vi "Filter VIs to Measure.vi"(8 "error in (no error)":errorcluster, 10 "VI Paths":path[](array[path]), 11 "Coverage Analyzer in":refnum<class "Coverage Analyzer.lvclass">) -> (0 "error out":errorcluster, 2 "Filtered VI Paths":path[](array[path]), 3 "Coverage Analyzer out":refnum<class "Coverage Analyzer.lvclass">)   [LabVIEW 2020, in "Coverage Analyzer.lvlib" / "Coverage Analyzer.lvclass"]
uses:
  Coverage Analyzer.lvclass
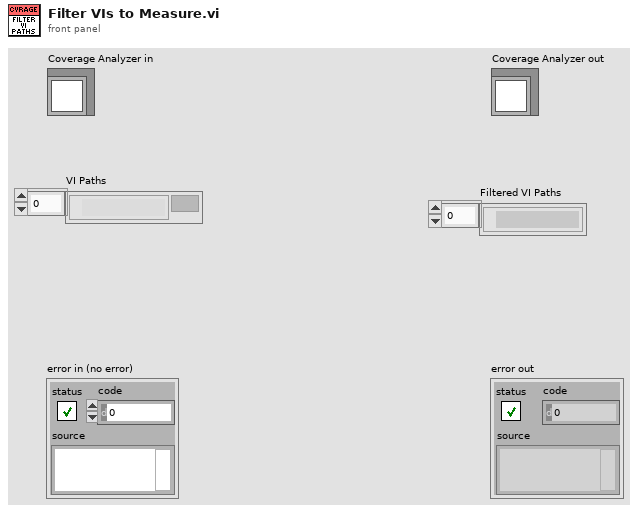
[diagram p1: front panel]
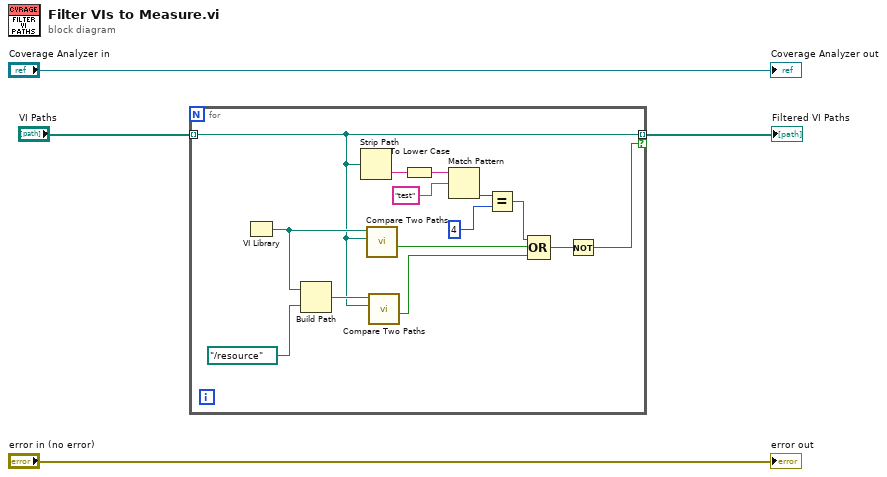
[diagram p0: block diagram]
diagram:
  n1 = for {
    tunnel: "VI Paths" -> [w11] mode=indexing
    tunnel: [w11] -> w2 mode=indexing if=w15
    n2 = VI Library() -> (path=w14:path)
    n3 = Build Path(base path=w14, name or relative path=path "../resource" ("search string")) -> (appended path=w17:path)
    n4 = Strip Path(path=w11) -> (name=w10:string)  [unwired: 1 out]
    n5 = call <vilib>:"Compare Two Paths.vi"("Path 2"=w11, "Path 1"=w14) -> ("Path 2 Relative to Path 1?"=w16:bool)  [unwired: 6 in, 3 out]
    n6 = call <vilib>:"Compare Two Paths.vi"("Path 2"=w11, "Path 1"=w17) -> ("Path 2 Relative to Path 1?"=w12:bool)  [unwired: 6 in, 3 out]
    n7 = To Lower Case(string=w10) -> (all lower case string=w9:string)
    n8 = Match Pattern(string=w9, regular expression="test") -> (offset past match=w7:i32)  [unwired: 1 in, 3 out]
    n9 = Equal?(x=w7, y=4) -> (x = y?=w5:bool)
    n10 = Compound Arithmetic op=OR(w5, w16, w12) -> (w13:bool)
    n11 = Not(x=w13) -> (.not. x?=w15:bool)
  }
  "Filtered VI Paths" <- w2
  "error out" <- "error in (no error)"
  "Coverage Analyzer out" <- "Coverage Analyzer in"
